vi "check source version Design Engine.vi"() -> (0 "continue running?":bool, 1 "Newer version available":bool, 2 "year":i32, 3 "application name":string, 4 "Application folder":path, 5 "time stamp":timestamp, 6 "error out":errorcluster, 7 "This version":timestamp, 11 "this version":path)   [LabVIEW 2011, in "Design Server.lvlib"]
uses:
  Design Server.lvlib
  version state.ctl
  <vilib>/Platform/browser.llb/Open URL in Default Browser (string).vi
panel:
  out "data":string
  out "version state":T1
  out "Connection":string
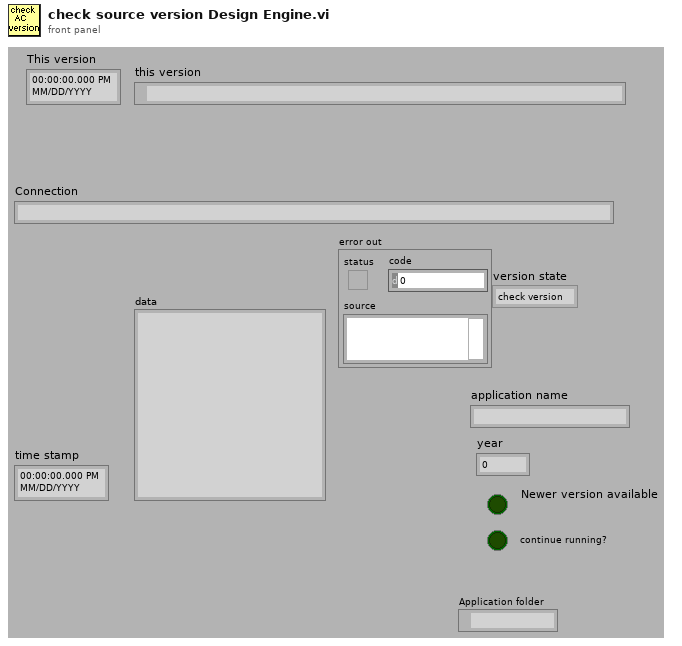
[diagram p1: front panel]
types:
  T1 = typedef "Design Server.lvlib/version state.ctl" = enum16{"check version", "prompt for update", "go to download", "accept license", "display copyright", "done"}
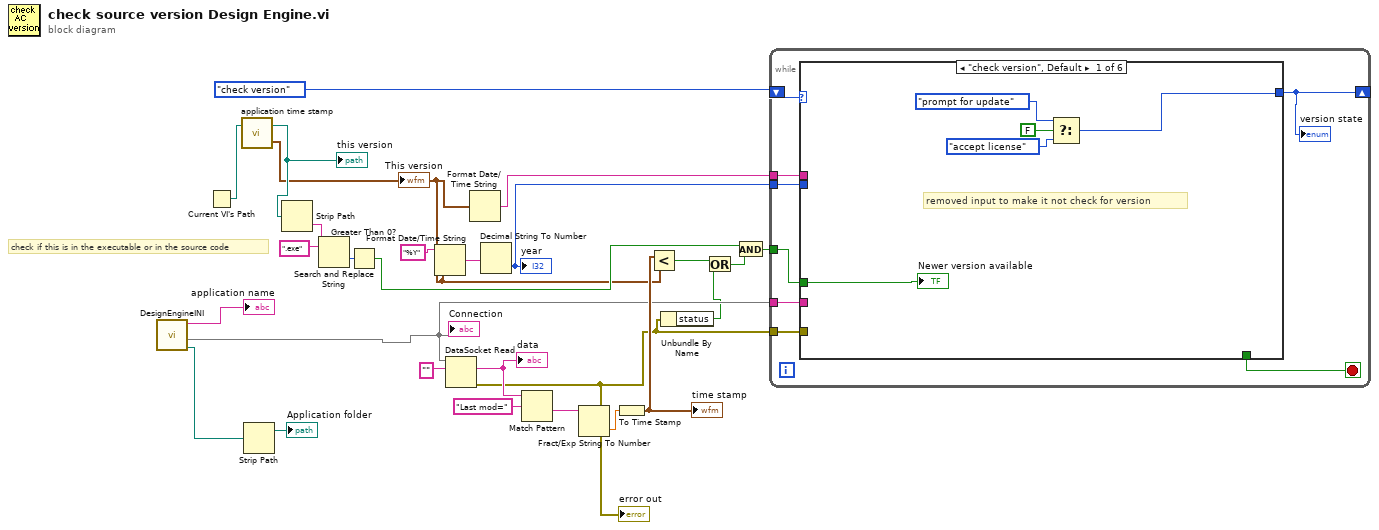
[diagram p0: block diagram]
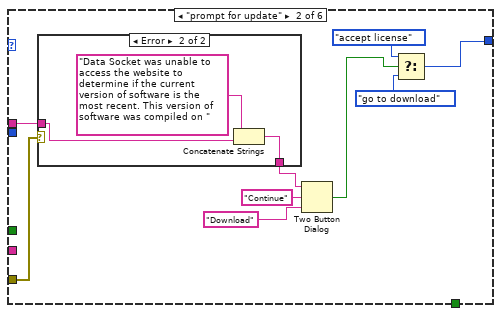
[diagram p2: hidden frame]
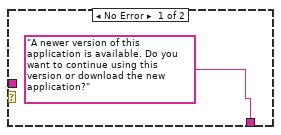
[diagram p3: hidden frame]
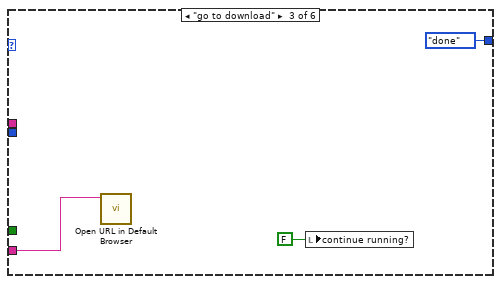
[diagram p4: hidden frame]
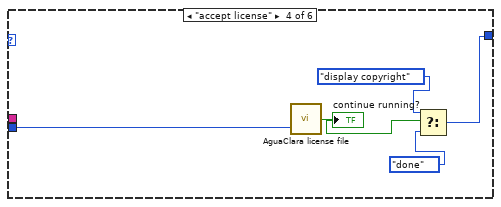
[diagram p5: hidden frame]
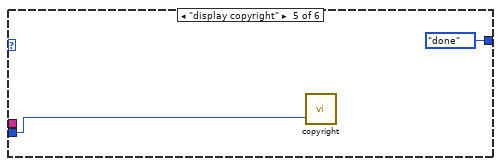
[diagram p6: hidden frame]
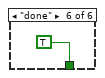
[diagram p7: hidden frame]
diagram:
  # "check if this is in the executable or in the source code"
  n1 = call "DesignEngineINI.vi"() -> ("Ini file path"=w11:path, 1:w12, "application name"=→"application name":string)  [unwired: 5 in]
  "Connection" <- w12
  n2 = Current VI's Path() -> (path=w3:path)
  n3 = call "application time stamp.vi"("VI Path"=w3) -> ("last mod"=w1:timestamp, "this version"=w2:path)  [unwired: 1 in]
  "This version" <- w1
  "this version" <- w2
  n4 = Strip Path(path=w11) -> (stripped path=→"Application folder":path)  [unwired: 1 out]
  n5 = Strip Path(path=w2) -> (name=w17:string)  [unwired: 1 out]
  n6 = Search and Replace String(input string=w17, search string=".exe") -> (offset past replacement=w18:i32)  [unwired: 6 in, 3 out]
  n7 = Greater Than 0?(x=w18) -> (x > 0?=w16:bool)
  n8 = Format Date/Time String(time format string (%c)="%Y", seconds (now)=w1) -> (date/time string=w5:string)  [unwired: 1 in]
  n9 = DataSocket Read(10:"" ("text"), 11:w12) -> (0:w6:errorcluster, 2:w22:string)  [unwired: 3 in, 5 out]
  "data" <- w22
  "error out" <- w6
  n10 = Format Date/Time String(seconds (now)=w1) -> (date/time string=w4:string)  [unwired: 2 in]
  n11 = Decimal String To Number(string=w5) -> (number=w21:i32)  [unwired: 2 in, 1 out]
  "year" <- w21
  n12 = Match Pattern(string=w22, regular expression="Last mod=") -> (after substring=w24:string)  [unwired: 1 in, 3 out]
  n13 = Fract/Exp String To Number(string=w24) -> (number=w25:dbl)  [unwired: 3 in, 1 out]
  n14 = To Time Stamp(1:w25) -> (0:w26:timestamp)
  "time stamp" <- w26
  n15 = Less?(x=w1, y=w26) -> (x < y?=w9:bool)
  n16 = Unbundle By Name(w6) -> ("status"=w7:bool)
  n17 = Or(x=w9, y=w7) -> (x .or. y?=w8:bool)
  n18 = And(x=w16, y=w8) -> (x .and. y?=w15:bool)
  n19 = while {
    shift-right: [w35] -> _
    shift-left: version_state."check version" ("version state") -> [w34]
    tunnel: w15 -> [w33]
    tunnel: w12 -> [w32]
    tunnel: w21 -> [w31]
    tunnel: w6 -> [w29]
    tunnel: w4 -> [w28]
    stop <- w30 stop-if-true
    n20 = case shown="\"check version\", Default" w34 {
      tunnel: [w40 w47 version_state."done" ("version state") w58 version_state."done" ("version state") _] -> w35
      tunnel: w33 -> [w37 _ _ _ _ _]
      tunnel: w32 -> [_ _ w54 _ _ _]
      tunnel: w31 -> [_ _ _ w61 w63 _]
      tunnel: [_ _ _ _ _ TRUE] -> w30
      tunnel: w29 -> [_ w46 _ _ _ _]
      tunnel: w28 -> [_ w41 _ _ _ _]
      frame "check version", Default {
        # "removed input to make it not check for version"
        n21 = Select(t=version_state."prompt for update" ("version state"), s=FALSE, f=version_state."accept license" ("version state")) -> (s? t:f=w40:T1)
        "Newer version available" <- w37
      }
      frame "prompt for update" {
        n22 = case shown="Error" w46 {
          tunnel: ["A newer version of this application is available. Do you want to continue using this version or download the new application?" ("message") w51] -> w42
          tunnel: w41 -> [_ w53]
          frame No Error {
          }
          frame Error {
            n23 = Concatenate Strings("Data Socket was unable to access the website to determine if the current version of software is the most recent. This version of software was compiled on " ("message"), w53) -> (w51:string)
          }
        }
        n24 = Two Button Dialog(message=w42, 1:"Download" ("F button name (\"Cancel\")"), 2:"Continue" ("T button name (\"OK\")")) -> (T button?=w43:bool)
        n25 = Select(t=version_state."accept license" ("version state"), s=w43, f=version_state."go to download" ("version state")) -> (s? t:f=w47:T1)
      }
      frame "go to download" {
        n26 = call-poly <vilib>:"Open URL in Default Browser.vi"("URL"=w54) -> ()  [unwired: 5 in, 2 out]
        n27 = local write "continue running?"(FALSE ("continue running?")) -> ()
      }
      frame "accept license" {
        n28 = call "AguaClara license file.vi"("year"=w61) -> ("Accepted"=w60:bool)  [unwired: 1 in]
        "continue running?" <- w60
        n29 = Select(t=version_state."display copyright" ("version state"), s=w60, f=version_state."done" ("version state")) -> (s? t:f=w58:T1)
      }
      frame "display copyright" {
        n30 = call "copyright.vi"("year"=w63) -> ()  [unwired: 3 in]
      }
      frame "done" {
      }
    }
    "version state" <- w35
  }
